vi "Load_Destinations.vi"(8 "error in (no error)":errorcluster, 11 "Installer in":refnum<class "Installer.lvclass">) -> (0 "error out":errorcluster, 3 "Installer out":refnum<class "Installer.lvclass">)   [LabVIEW 2020, in "Installer.lvclass"]
uses:
  <vilib>/AppBuilder/IB_Classes/Installer/Installer.lvclass
  <vilib>/AppBuilder/IB_Classes/Installer/Installer.lvclass/Installer.ctl
  <vilib>/AppBuilder/IB_Classes/Destination/IB_Destination.lvclass
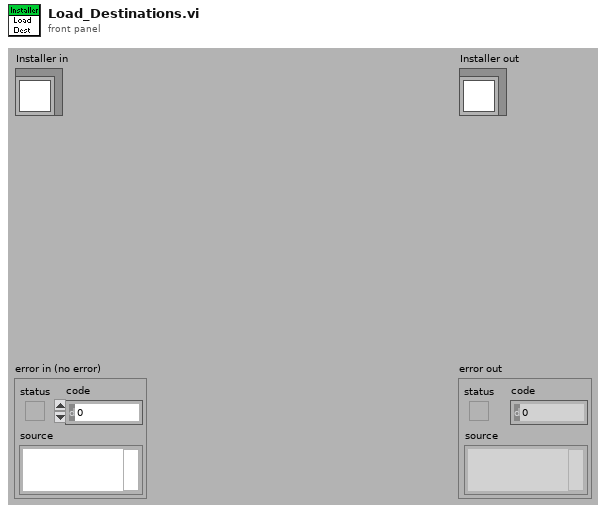
[diagram p1: front panel]
types:
  T1 = typedef "ItemRef.ctl" = u64
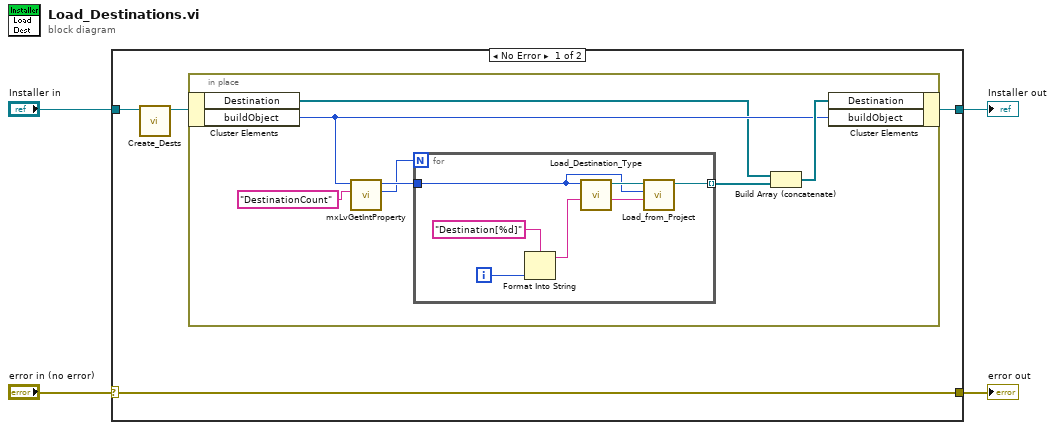
[diagram p0: block diagram]
diagram:
  n1 = case shown="No Error" "error in (no error)" {
    selector: "error in (no error)" -> [w8 w24]
    tunnel: [w8 w24] -> w3
    tunnel: [w5 w23] -> w1
    tunnel: "Installer in" -> [w7 w23]
    frame No Error {
      n2 = call-dynamic "Create_Dests.vi"("Class in"=w7) -> ("Class out"=w6:refnum<class "Installer.lvclass">)  [unwired: 1 in, 9 out]
      n3 = in-place {
        n4 = in-place-cluster #1(w6) -> ("Destination"=w9:refnum<class "IB_Destination.lvclass">[], "buildObject"=w10:T1)
        n5 = call <resource>:"mxLvGetIntProperty.vi"("Tag"="DestinationCount", "Item"=w10) -> ("Value"=w14:i32, "Item"=w15:T1)  [unwired: 1 in, 7 out]
        n6 = for {
          N: w14 -> [_]
          tunnel: w15 -> [w21]
          tunnel: [w20] -> w12 mode=indexing
          i -> [w18]
          n7 = Format Into String(format string="Destination[%d]", w18) -> (resulting string=w17:string)  [unwired: 2 in, 1 out]
          n8 = call <vilib>:"Load_Destination_Type.vi"("index"=w17, "buildObject"=w21) -> ("index out"=w16:string, "IB_Destination out"=w22:refnum<class "IB_Destination.lvclass">)  [unwired: 1 in, 7 out]
          n9 = call-dynamic "Load_from_Project.vi"("index"=w16, "buildObject"=w21, "IB_Destination.lvclass"=w22) -> ("IB_Destination out"=w20:refnum<class "IB_Destination.lvclass">)  [unwired: 1 in, 7 out]
        }
        n10 = Build Array (concatenate)(w9, w12) -> (w11:refnum<class "IB_Destination.lvclass">[])
        n11 = in-place-cluster #1("Destination"=w11, "buildObject"=w10) -> (w5:refnum<class "Installer.lvclass">)
      }
    }
    frame Error {
    }
  }
  "error out" <- w3
  "Installer out" <- w1
